vi "TCP AK-LNI Befehl Senden.vi"(6 "Don't Care Char (Leerz.)":string=" ", 7 "Kanalnummer (K0)":u8 max=99 step=1, 8 "Fehler (Eingang)":errorcluster, 9 "Daten":string[](array[string]), 10 "Befehl (4 Zeichen)":string, 11 "Verbindungs-ID":refnum<k5>) -> (0 "Fehler (Ausgang)":errorcluster, 3 "Verbindungs-ID":refnum<k5>)   [LabVIEW 2020, in "Linearisierung v2.lvlib" / "Gasteiler.lvlib" / "AK Komm Gasteiler.lvlib"]
doc: "Bereitet ein vollständiges Befehls-Telegramm aus folgenden Eingangsdaten auf:\n\n\"Befehl\": immer vier ASCII-Zeichen (Großbuchstaben)\n\n\"Daten\": 1D-Array aus ASCII-String nach Vorgabe des Befehls.\n\n\"Kanalnummer\" (U8) kann Werte von 0 bis 255 annehmen. Standardwert ist 0.\n\n\"Don't Care Char\": druckbares ASCII-Zeichen, Standard Leerzeichen"
uses:
  AK Komm Gasteiler.lvlib
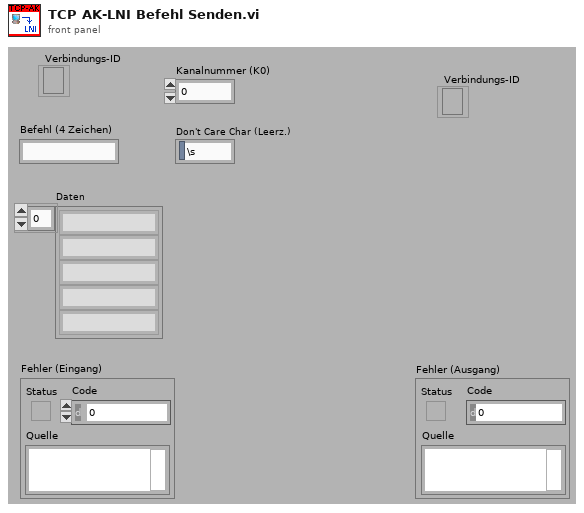
[diagram p1: front panel]
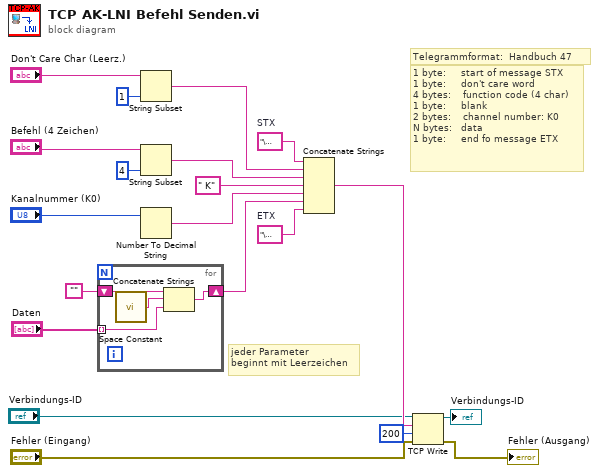
[diagram p0: block diagram]
diagram:
  w16 = "\u0003"  # ETX
  w15 = "\u0002"  # STX
  # "jeder Parameter\nbeginnt mit Leerzeichen"
  # "Telegrammformat:  Handbuch 47"
  # "1 byte:     start of message STX\n1 byte:     don't care word\n4 bytes:    function code (4 char)\n1 byte:     blank\n2 bytes:    channel number: K0\nN bytes:   data\n1 byte:     end fo message ETX"
  n1 = for {
    tunnel: "Daten" -> [w22] mode=indexing
    shift-right: [w21] -> w8
    shift-left: "" -> [w24]
    n2 = call <vilib>:"Space Constant.vi"() -> ("String"=w23:string)
    n3 = Concatenate Strings(w24, w23, w22) -> (w21:string)
  }
  n4 = String Subset(string="Don't Care Char (Leerz.)", length (rest)=1 ("Länge (Rest)")) -> (substring=w4:string)  [unwired: 1 in]
  n5 = String Subset(string="Befehl (4 Zeichen)", length (rest)=4 ("Länge (Rest)")) -> (substring=w14:string)  [unwired: 1 in]
  n6 = Number To Decimal String(number="Kanalnummer (K0)") -> (decimal integer string=w12:string)  [unwired: 1 in]
  n7 = Concatenate Strings(w15, w4, w14, " K" ("String"), w12, w8, w16) -> (w13:string)
  n8 = TCP Write(connection ID="Verbindungs-ID", data in=w13, error in (no error)="Fehler (Eingang)", 9:200 ("Timeout in ms (25000)")) -> (connection ID out=→"Verbindungs-ID":refnum<k5>, error out=→"Fehler (Ausgang)":errorcluster)  [unwired: 1 out]
